vi "Test - helloDqmhWorldModule - Do Something Else and Wait for Reply 1.vi"(8 "error in":errorcluster) -> (0 "error out":errorcluster)   [LabVIEW 2023]
doc: "_____\nCreated using DQMH Event Scripter 7.0.0.1280."
uses:
  <vilib>/addons/_JKI Toolkits/Caraya/classes/Assert/Assert Almost Equal_Float.vi
  Libraries/helloDqmhWorldModule/helloDqmhWorldModule.lvlib
  <vilib>/addons/_JKI Toolkits/Caraya/classes/Test/Test.lvclass
  <vilib>/addons/_JKI Toolkits/Caraya/classes/Assert/Assert.lvclass
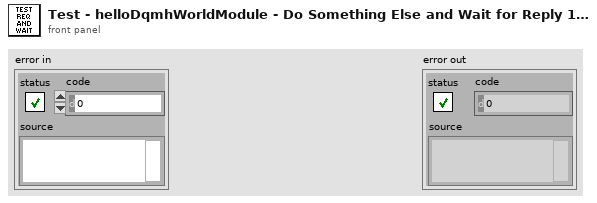
[diagram p1: front panel]
types:
  T1 = typedef "helloDqmhWorldModule.lvlib/Do Something Else and Wait (Reply Payload)--cluster.ctl" = cluster{"Value":dbl, "error":errorcluster}
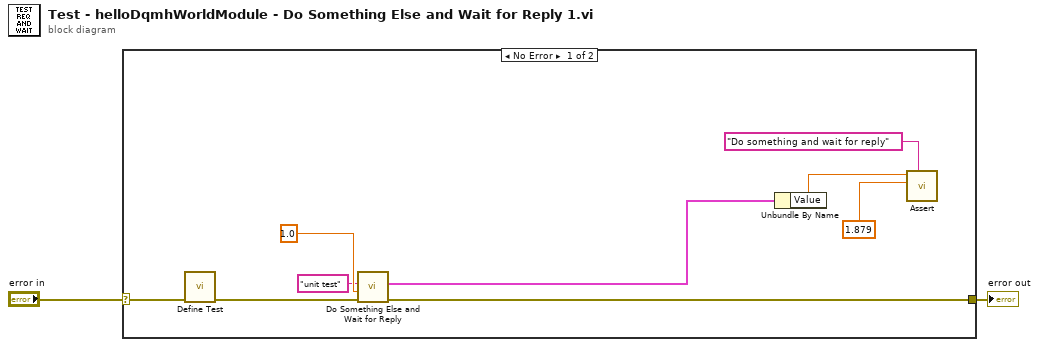
[diagram p0: block diagram]
diagram:
  n1 = case shown="No Error" "error in" {
    selector: "error in" -> [w7 w12]
    tunnel: [w11 w12] -> w1
    frame No Error {
      n2 = call <vilib>:"Define Test.vi"("error in (no error)"=w7) -> ("error out"=w6:errorcluster)  [unwired: 9 in, 1 out]
      n3 = call "Do Something Else and Wait for Reply.vi"("error in"=w6, "X"=1.0, "Do Something Else Message"="unit test") -> ("error out"=w11:errorcluster, "Reply Payload"=w10:T1)  [unwired: 6 in, 1 out]
      n4 = Unbundle By Name(w10) -> ("Value"=w4:dbl)
      n5 = call-poly <vilib>:"Assert.vi"("Label"="Do something and wait for reply" ("Label (VI Title)"), "Y"=1.879 ("Value"), "X"=w4) -> ()  [unwired: 7 in, 2 out]
    }
    frame Error {
    }
  }
  "error out" <- w1
